vi "JSON Tree to Topology.vi"(8 "error in (no error)":errorcluster, 11 "JSON Array":variant) -> (0 "error out":errorcluster, 2 "Topology":T1)   [LabVIEW 2015, in "SLSC Switch.lvlib" / "SLSC Switch.lvclass"]
uses:
  SLSC Switch.lvclass
  Controls/JSON.Topology.ctl
  Controls/JSON.InitialState.ctl
  Controls/JSON.ChannelList.ctl
  Controls/JSON.ConnectionList.ctl
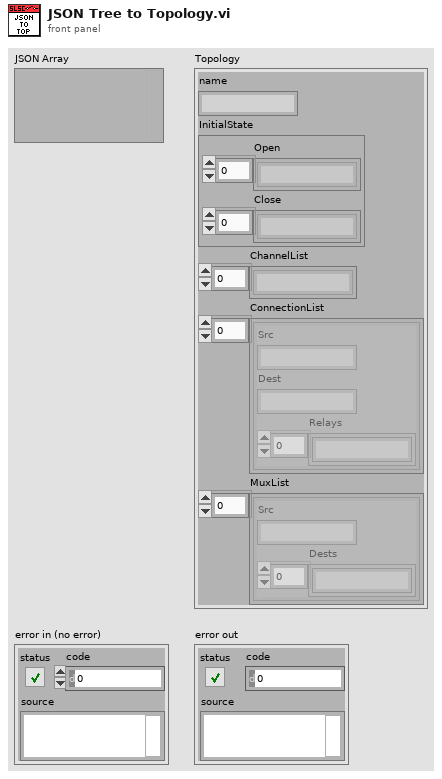
[diagram p1: front panel]
types:
  T1 = typedef "SLSC Switch.lvlib/SLSC Switch.lvclass/JSON.Topology.ctl" = cluster{"name":string, "InitialState":T2, "ChannelList":T3, "ConnectionList":T4[], "MuxList":cluster{"Src":string, "Dests":string[]}[]}
  T2 = typedef "SLSC Switch.lvlib/SLSC Switch.lvclass/JSON.InitialState.ctl" = cluster{"Open":string[], "Close":string[]}
  T3 = typedef "SLSC Switch.lvlib/SLSC Switch.lvclass/JSON.ChannelList.ctl" = string[]
  T4 = typedef "SLSC Switch.lvlib/SLSC Switch.lvclass/JSON.ConnectionList.ctl" = cluster{"Src":string, "Dest":string, "Relays":string[]}
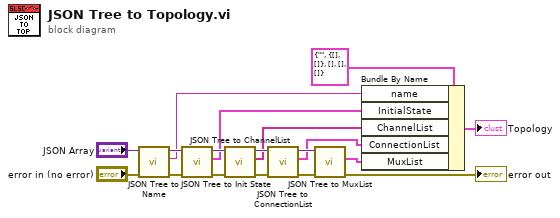
[diagram p0: block diagram]
diagram:
  n1 = call "JSON Tree to Name.vi"("error in (no error)"="error in (no error)", "JSON Array"="JSON Array") -> ("error out"=w16:errorcluster, "Name"=w7:string, "JSON Tree Out Passthrough"=w10:variant)  [unwired: 7 in]
  n2 = call "JSON Tree to Init State.vi"("error in (no error)"=w16, "JSON Tree Out Passthrough"=w10) -> ("error out"=w17:errorcluster, "Initial State"=w6:T2, "JSON Tree Out"=w11:variant)  [unwired: 7 in]
  n3 = call "JSON Tree to ChannelList.vi"("error in (no error)"=w17, "JSON Tree Out"=w11) -> ("error out"=w13:errorcluster, "ChannelList"=w3:T3, "JSON Tree Out Passthrough"=w12:variant)  [unwired: 7 in]
  n4 = call "JSON Tree to ConnectionList.vi"("error in (no error)"=w13, "JSON Array"=w12) -> ("error out"=w18:errorcluster, "ConnectionList"=w5:T4[], "JSON Tree Passthrough (JSON Array)"=w14:variant)  [unwired: 7 in]
  n5 = call "JSON Tree to MuxList.vi"("error in (no error)"=w18, "JSON Array"=w14) -> ("error out"=→"error out":errorcluster, "MuxList"=w4:cluster{"Src":string, "Dests":string[]}[])  [unwired: 7 in, 1 out]
  n6 = Bundle By Name(cluster=T1 {"name"="", "InitialState"={"Open"=[], "Close"=[]}, "ChannelList"=[], "ConnectionList"=[], "MuxList"=[]} ("Topology"), "name"=w7, "InitialState"=w6, "ChannelList"=w3, "ConnectionList"=w5, "MuxList"=w4) -> (→"Topology":T1)
